vi "Shooter.vi"(1 "FrontMotorIn":dbl, 2 "Control Mode":T1=enum."Unchanged / Invalid", 3 "RearMotorIn":dbl) -> ()   [LabVIEW 2016]
uses:
  <vilib>/Rock Robotics/WPI/ThirdParty/CanMotor/TalonSRX/WPI_CANTalonSRX_APIControlMode.ctl
  <vilib>/Rock Robotics/WPI/ThirdParty/CanMotor/TalonSRX/WPI_CANTalonSRX_APIFeedbackSelect.ctl
panel:
  out "Applied Throttle":dbl
  out "Speed Closed Loop Plots Rear":cluster{dbl, "Sensor Velocity":dbl}(graph)
  out "Speed Closed Loop Plots Front":cluster{dbl, "Sensor Velocity":dbl}(graph)
  out "Encoder Velocity Rear":dbl
  out "Encoder Velocity Front":dbl
  in  "Ramp Rate Rear":dbl format="%#_13g"
  in  "I Zone Rear":dbl format="%#_13g"
  in  "F Rear":dbl=0.03 format="%#_13g"
  in  "D Rear":dbl format="%#_13g"
  in  "I Rear":dbl=0.0002 format="%#_13g"
  in  "P Rear":dbl format="%#_13g"
  in  "Ramp Rate Front":dbl format="%#_13g"
  in  "I Zone Front":dbl format="%#_13g"
  in  "F Front":dbl=0.03 format="%#_13g"
  in  "D Front":dbl format="%#_13g"
  in  "I Front":dbl=0.0002 format="%#_13g"
  in  "P Front":dbl format="%#_13g"
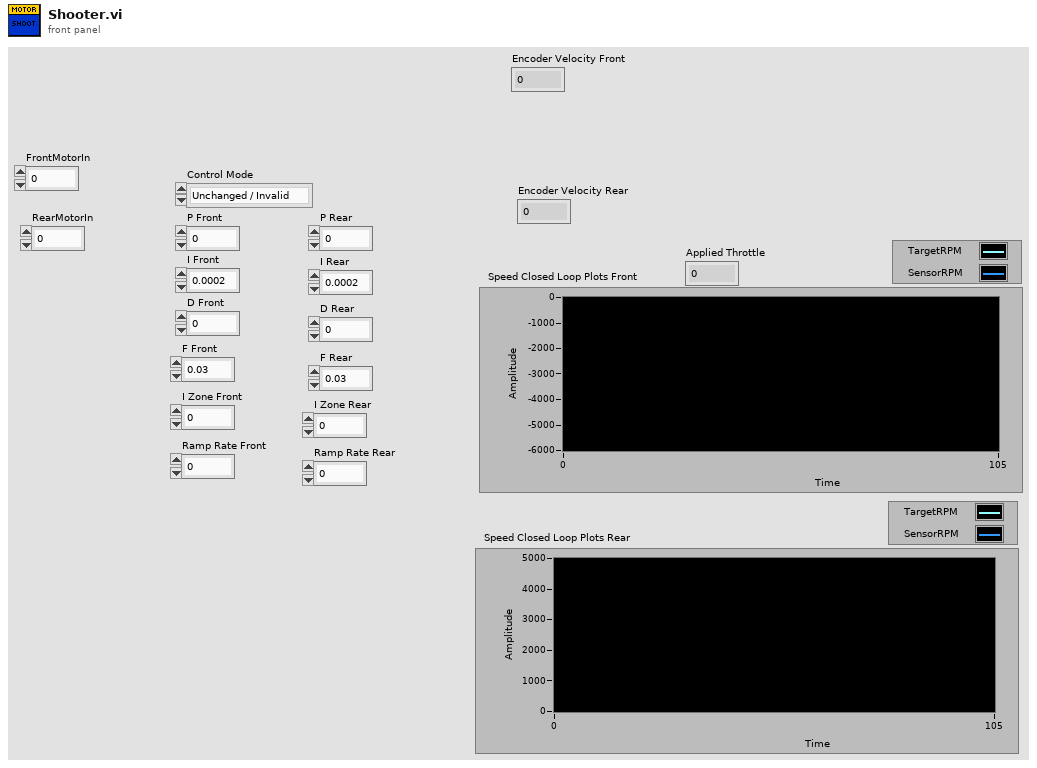
[diagram p1: front panel]
types:
  T1 = typedef "WPI_CANTalonSRX_APIControlMode.ctl" = enum8{"Percent VBus", "Speed", "Position", "Slave", "Unchanged / Invalid", "Voltage Compensation", "Current", "Motion Profile", "Motion Magic"}
  T2 = typedef "WPI_MotorControlDeviceRef.ctl" = cluster{"DeviceStatus":errorcluster, "Type":T3, "PWM":cluster{"PWM Channel":T4, "DeadBand":T5}, "CAN":cluster{"Device Number":u8, "SetOutput VI Ref":variant, "GetOutput VI Ref":variant, "Enable VI Ref":variant, "Disable VI Ref":variant, "Data":variant}, "Invert":bool}
  T3 = typedef "WPI_MotorControlType.ctl" = enum16{"PWM", "CAN"}
  T4 = typedef "FPGA_DIOPWMChannel.ctl" = enum8{"PWM 0", "PWM 1", "PWM 2", "PWM 3", "PWM 4", "PWM 5", "PWM 6", "PWM 7", "PWM 8", "PWM 9", "PWM MXP 0", "PWM MXP 1", "PWM MXP 2", "PWM MXP 3", "PWM MXP 4", "PWM MXP 5", "PWM MXP 6", "PWM MXP 7", "PWM MXP 8", "PWM MXP 9", "Invalid"}
  T5 = typedef "WPI_PWMDeadband.ctl" = cluster{"Name":string, "maxPositivePwm":i32, "minPositivePwm":i32, "centerPwm":i32, "maxNegativePwm":i32, "minNegativePwm":i32, "angularRange":u16}
  T6 = typedef "WPI_CANTalonSRX_GlobalStatus.ctl" = cluster{"Applied Throttle":dbl, "Module Enabled":bool, "CAN Error":errorcluster, "Closed Loop Error":dbl, "Forward Limit Switch Closed":bool, "Reverse Limit Switch Closed":bool, "Sensor Position":dbl, "Sensor Velocity":dbl, "Current":dbl, "Sticky Fault - Over Temp":bool, "Sticky Fault - Under Voltage":bool, "Sticky Fault - Forward Limit":bool, "Sticky Fault - Reverse Limit":bool, "Sticky Fault - Forward Soft Limit":bool, "Sticky Fault - Reverse Soft Limit":bool, "Brake is Enabled":bool, "Encoder Position":dbl, "Encoder Velocity":dbl, "Encoder Index Count":dbl, "Encoder A Pin State":bool, "Encoder B Pin State":bool, "Encoder Index Pin State":bool, "Analog In":dbl, "Analog In Velocity":dbl, "Temperature (C)":dbl, "Battery Voltage":dbl, "Control 5 Is Supported":bool, "Current Profile Slot Select":dbl, "Pos Div 8":bool, "Vel Div 4":bool, "Pulse Width Position":i32, "Pulse Width Velocity":i32, "Pulse Width Rise To Rise (us)":i32, "Pulse Width Rise To Fall (us)":i32, "Mot Prof Active Is Under Run":bool, "Mot Prof Active Has Under Run":bool, "Mot Prof Active Is Last":bool, "Mot Prof Active Velocity Only":bool, "Mot Prof Active Is Valid":bool, "Mot Prof Buffer Is Full":bool, "Mot Prof Active Profile Slot Select":i32, "Mot Prof NextID":i32, "Mot Prof Count":i32, "Mot Prof Active Velocity":dbl, "Mot Prof Active Position":dbl, "Mot Prof Output Enable":i32, "UsageFrame":u32, "Motion Magic Active Trajectory":cluster{"Velocity":dbl, "Position":dbl}}
  T7 = typedef "WPI_CANTalonSRX_APIFeedbackSelect.ctl" = enum16{"Digital Quadrature Encoder", "Analog Potentiometer", "Analog Encoder", "Count on Quad-A (Rising-Edge)", "Count on Quad-A (Falling-Edge)", "CTR Magnetic Enc (Absolute)", "CTR Magnetic Enc (Relative)", "Pulse Width"}
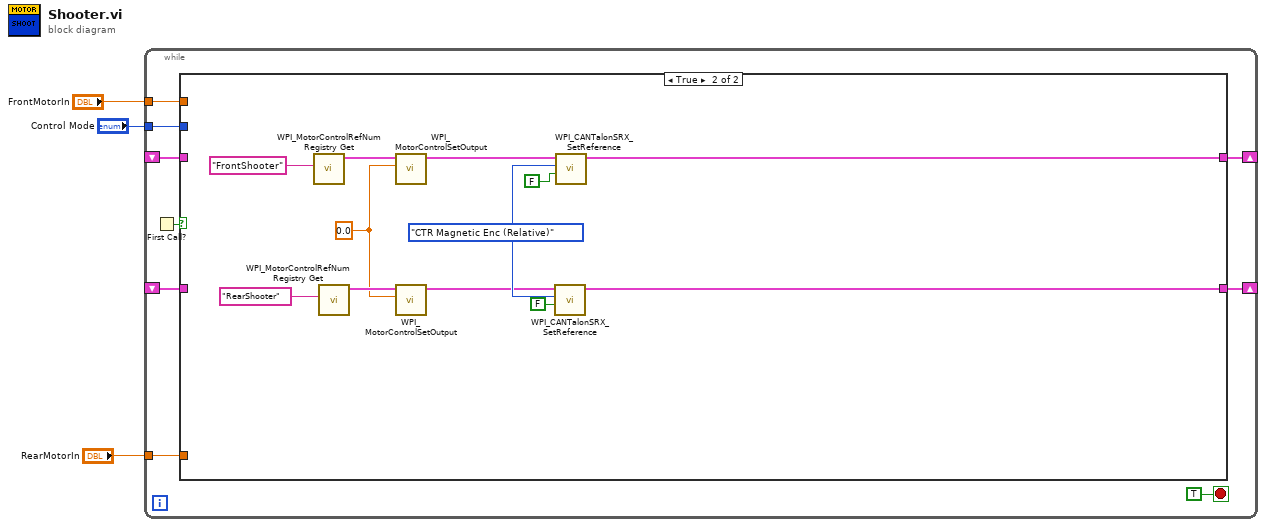
[diagram p0: block diagram]
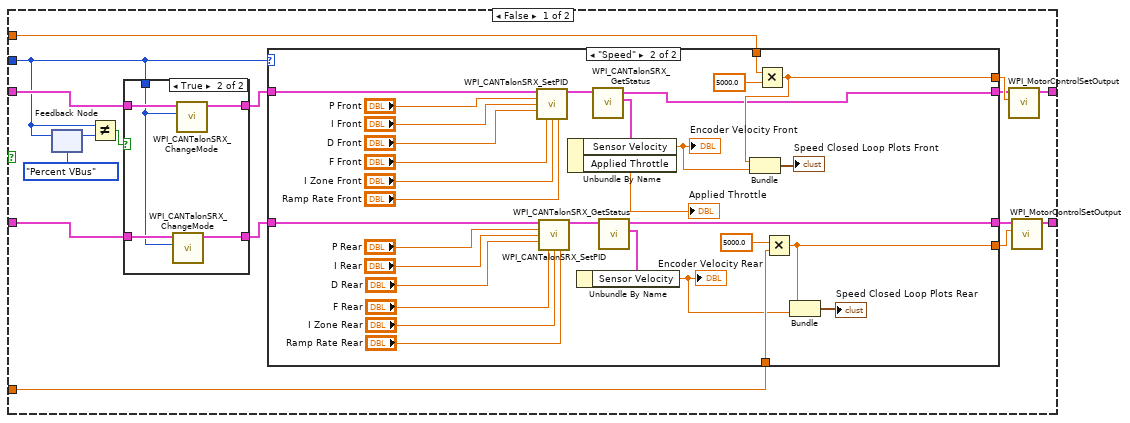
[diagram p2: hidden frame]
diagram:
  n1 = while {
    shift-right: [w9] -> _
    shift-left: _ -> [w10]
    shift-right: [w8] -> _
    shift-left: _ -> [w7]
    tunnel: "Control Mode" -> [w6]
    tunnel: "FrontMotorIn" -> [w5]
    tunnel: "RearMotorIn" -> [w4]
    stop <- TRUE stop-if-true
    n2 = First Call?() -> (First Call?: T/F=w11:bool)
    n3 = case shown="True" w11 {
      tunnel: w10 -> [w28 _]
      tunnel: [w15 w73] -> w9
      tunnel: [w16 w74] -> w8
      tunnel: w7 -> [w25 _]
      tunnel: w6 -> [w22 _]
      tunnel: w5 -> [w24 _]
      tunnel: w4 -> [w23 _]
      frame False {
        n4 = feedback #1(WPI_CANTalonSRX_APIControlMode."Percent VBus" ("Control Mode")) -> (w21:T1)
        n5 = feedback-in #1(w22) -> ()
        n6 = Not Equal?(x=w22, y=w21) -> (x != y?=w19:bool)
        n7 = case shown="True" w19 {
          tunnel: w28 -> [w30 w33]
          tunnel: [w30 w32] -> w27
          tunnel: [w29 w34] -> w26
          tunnel: w25 -> [w29 w35]
          tunnel: w22 -> [_ w31]
          frame False {
          }
          frame True {
            n8 = call <vilib>:"WPI_CANTalonSRX_ChangeMode.vi"("Control Mode"=w31, "CAN Talon SRX Ref"=w35) -> ("CAN Talon SRX Ref"=w34:T2)  [unwired: 8 in, 1 out]
            n9 = call <vilib>:"WPI_CANTalonSRX_ChangeMode.vi"("Control Mode"=w31, "CAN Talon SRX Ref"=w33) -> ("CAN Talon SRX Ref"=w32:T2)  [unwired: 8 in, 1 out]
          }
        }
        n10 = case shown="\"Speed\"" w22 {
          tunnel: w27 -> [w39 w58]
          tunnel: [w39 w41] -> w17
          tunnel: w26 -> [w36 w57]
          tunnel: [w36 w52] -> w14
          tunnel: w24 -> [w38 w51]
          tunnel: w23 -> [w37 w48]
          tunnel: [w37 w47] -> w13
          tunnel: [w38 w44] -> w18
          frame "Percent VBus", Default {
          }
          frame "Speed" {
            n11 = call <vilib>:"WPI_CANTalonSRX_SetPID.vi"("CAN Talon SRX Ref"=w58, "P"="P Front", "I"="I Front", "D"="D Front", "F"="F Front", "I Zone"="I Zone Front", "Ramp Rate"="Ramp Rate Front") -> ("CAN Talon SRX Ref"=w56:T2)  [unwired: 7 in, 1 out]
            n12 = call <vilib>:"WPI_CANTalonSRX_SetPID.vi"("CAN Talon SRX Ref"=w57, "P"="P Rear", "I"="I Rear", "D"="D Rear", "F"="F Rear", "I Zone"="I Zone Rear", "Ramp Rate"="Ramp Rate Rear") -> ("CAN Talon SRX Ref"=w53:T2)  [unwired: 7 in, 1 out]
            n13 = call <vilib>:"WPI_CANTalonSRX_GetStatus.vi"("CAN Talon SRX Ref"=w56) -> ("Talon SRX Status"=w55:T6, "CAN Talon SRX Ref"=w41:T2)  [unwired: 8 in, 1 out]
            n14 = Unbundle By Name(w55) -> ("Sensor Velocity"=w43:dbl, "Applied Throttle"=→"Applied Throttle":dbl)
            "Encoder Velocity Front" <- w43
            n15 = call <vilib>:"WPI_CANTalonSRX_GetStatus.vi"("CAN Talon SRX Ref"=w53) -> ("Talon SRX Status"=w54:T6, "CAN Talon SRX Ref"=w52:T2)  [unwired: 8 in, 1 out]
            n16 = Unbundle By Name(w54) -> ("Sensor Velocity"=w46:dbl)
            "Encoder Velocity Rear" <- w46
            n17 = Multiply(x=w51, y=5000.0) -> (x*y=w44:dbl)
            n18 = Bundle(w44, "Sensor Velocity"=w43) -> (→"Speed Closed Loop Plots Front":cluster{dbl, "Sensor Velocity":dbl})  [unwired: 1 in]
            n19 = Multiply(x=5000.0 ("y"), y=w48) -> (x*y=w47:dbl)
            n20 = Bundle(w47, "Sensor Velocity"=w46) -> (→"Speed Closed Loop Plots Rear":cluster{dbl, "Sensor Velocity":dbl})  [unwired: 1 in]
          }
        }
        n21 = call <vilib>:"WPI_MotorControlSetOutput.vi"("Output"=w18, "MotorControlDevRef"=w17) -> ("MotorControlDevRef"=w15:T2)  [unwired: 7 in, 2 out]
        n22 = call <vilib>:"WPI_MotorControlSetOutput.vi"("Output"=w13, "MotorControlDevRef"=w14) -> ("MotorControlDevRef"=w16:T2)  [unwired: 7 in, 2 out]
      }
      frame True {
        w77 = WPI_CANTalonSRX_APIFeedbackSelect."CTR Magnetic Enc (Relative)" ("Feedback Reference")
        w78 = 0.0 ("Output")
        n23 = call <vilib>:"WPI_MotorControlRefNum Registry Get.vi"("refnum name"="FrontShooter") -> ("MotorControlDevRef"=w80:T2)  [unwired: 9 in, 1 out]
        n24 = call <vilib>:"WPI_MotorControlRefNum Registry Get.vi"("refnum name"="RearShooter") -> ("MotorControlDevRef"=w79:T2)  [unwired: 9 in, 1 out]
        n25 = call <vilib>:"WPI_MotorControlSetOutput.vi"("Output"=w78, "MotorControlDevRef"=w80) -> ("MotorControlDevRef"=w76:T2)  [unwired: 7 in, 2 out]
        n26 = call <vilib>:"WPI_MotorControlSetOutput.vi"("Output"=w78, "MotorControlDevRef"=w79) -> ("MotorControlDevRef"=w75:T2)  [unwired: 7 in, 2 out]
        n27 = call <vilib>:"WPI_CANTalonSRX_SetReference.vi"("Reverse Feedback Sensor"=FALSE, "Feedback Reference"=w77, "CAN Talon SRX Ref"=w75) -> ("CAN Talon SRX Ref"=w74:T2)  [unwired: 7 in, 1 out]
        n28 = call <vilib>:"WPI_CANTalonSRX_SetReference.vi"("Reverse Feedback Sensor"=FALSE, "Feedback Reference"=w77, "CAN Talon SRX Ref"=w76) -> ("CAN Talon SRX Ref"=w73:T2)  [unwired: 7 in, 1 out]
      }
    }
  }
